vi "templates analysis BODY data keys.vi"(9 "Template Keys":T1, 10 "HTM Keys":T1) -> (2 "HTM Keys":T1)   [LabVIEW 2011]
uses:
  Addons/internet/utils/keyedarr.llb/Keyed Array.ctl
  Addons/internet/utils/strutil.llb/Case Matching.ctl
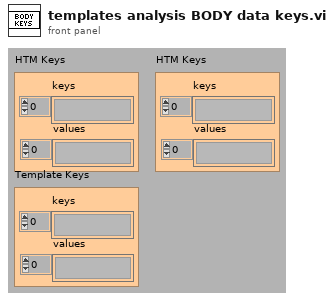
[diagram p1: front panel]
types:
  T1 = typedef "Keyed Array.ctl" = cluster{"keys":string[], "values":string[]}
  T2 = typedef "Case Matching.ctl" = enum16{"a != A", "a == A", "system"}
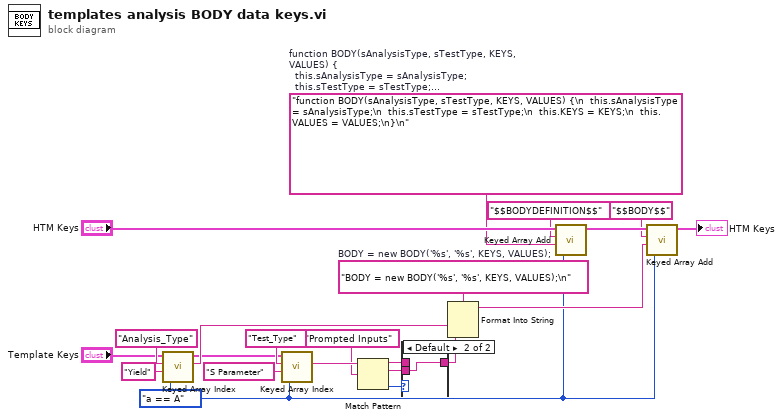
[diagram p0: block diagram]
diagram:
  w1 = Case_Matching."a == A" ("case matching (sensitive)")
  w16 = "BODY = new BODY('%s', '%s', KEYS, VALUES);\n"  # BODY = new BODY('%s', '%s', KEYS, VALUES);
  w20 = "function BODY(sAnalysisType, sTestType, KEYS, VALUES) {\n  this.sAnalysisType = sAnalysisType;\n  this.sTestType = sTestType;\n  this.KEYS = KEYS;\n  this.VALUES = VALUES;\n}\n"  # function BODY(sAnalysisType, sTestType, KEYS, VALUES) {   this.sAnalysisType = sAnalysisType;   this.sTestType = sTestType;   this.KEYS = KEYS;   this.VALUES = VALUES; }
  n1 = call "Keyed Array Index.vi"("case matching (sensitive)"=w1, "default value"="Yield" ("key"), "key"="Analysis_Type", "array in"="Template Keys") -> ("value"=w4:string, "duplicate array"=w3:T1)  [unwired: 2 out]
  n2 = call "Keyed Array Index.vi"("case matching (sensitive)"=w1, "default value"="S Parameter" ("key"), "key"="Test_Type", "array in"=w3) -> ("value"=w12:string)  [unwired: 3 out]
  n3 = Match Pattern(string=w12, regular expression="Prompted Inputs") -> (before substring=w9:string, match substring=w7:string, offset past match=w10:i32)  [unwired: 2 out]
  n4 = case shown="Default" w10 {
    tunnel: w9 -> [w23 _]
    tunnel: [w23 w24] -> w8
    tunnel: w7 -> [_ w24]
    frame -1 {
    }
    frame Default {
    }
  }
  n5 = Format Into String(format string=w16, w4, w8) -> (resulting string=w14:string)  [unwired: 2 in, 1 out]
  n6 = call "Keyed Array Add.vi"("case matching (sensitive)"=w1, "value"=w20, "key"="$$BODYDEFINITION$$", "array in"="HTM Keys") -> ("array out"=w19:T1)  [unwired: 3 out]
  n7 = call "Keyed Array Add.vi"("case matching (sensitive)"=w1, "value"=w14, "key"="$$BODY$$", "array in"=w19) -> ("array out"=→"HTM Keys":T1)  [unwired: 3 out]
